vi "Read Spot Measurement.vi"(7 "Enable Channel 1 to 2":bool, 8 "error in (no error)":errorcluster, 9 "Measurement Mode (0:Voltage)":enum16{"Voltage", "Current", "Resistance"}(ring), 10 "Channel List ({Channel1})":i32[](array[ring])=[0] items=["Channel 1", "Channel 2"], 11 "VISA resource name":refnum<visa-resource-name>) -> (0 "error out":errorcluster, 2 "Measurement Result":dbl, 3 "VISA resource name out":refnum<visa-resource-name>)   [LabVIEW 2023, in "Agilent B2900 Series.lvlib"]
doc: "Reads the measurement result data after it executes a spot measurement (one-shot measurement)"
uses:
  Agilent B2900 Series.lvlib
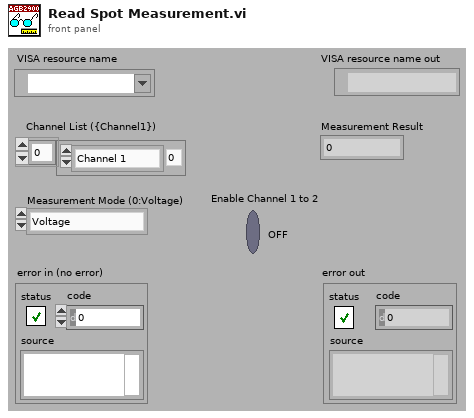
[diagram p1: front panel]
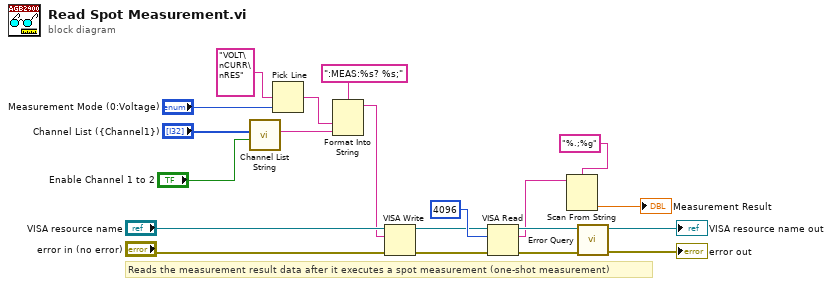
[diagram p0: block diagram]
diagram:
  # "Reads the measurement result data after it executes a spot measurement (one-shot measurement)"
  n1 = call "Channel List String.vi"("Enable Channel 1 to 2"="Enable Channel 1 to 2", "Channel List ({Channel1})"="Channel List ({Channel1})") -> ("Channel List Command String"=w5:string)  [unwired: 9 in]
  n2 = Pick Line(multi-line string="VOLT\nCURR\nRES", line index="Measurement Mode (0:Voltage)") -> (output string=w6:string)  [unwired: 1 in]
  n3 = Format Into String(format string=":MEAS:%s? %s;", w6, w5) -> (resulting string=w9:string)  [unwired: 2 in, 1 out]
  n4 = VISA Write(VISA resource name="VISA resource name", write buffer=w9, error in (no error)="error in (no error)") -> (VISA resource name out=w17:refnum<visa-resource-name>, error out=w16:errorcluster)  [unwired: 1 out]
  n5 = VISA Read(VISA resource name=w17, byte count=u32 4096, error in (no error)=w16) -> (VISA resource name out=w15:refnum<visa-resource-name>, read buffer=w2:string, error out=w14:errorcluster)  [unwired: 1 out]
  n6 = Scan From String(format string="%.;%g", input string=w2) -> (output 1=→"Measurement Result":dbl)  [unwired: 3 in, 3 out]
  n7 = call "Error Query.vi"("error in (no error)"=w14, "VISA resource name"=w15) -> ("error out"=→"error out":errorcluster, "VISA resource name out"=→"VISA resource name out":refnum<visa-resource-name>)  [unwired: 6 in, 2 out]
